vi "fft_tmp.vi"() -> ()   [LabVIEW 2014]
uses:
  <vilib>/express/express analysis/Spectral/Block/exnSpectralBlock spectral measurements peak poly.vi
  <vilib>/express/express analysis/Spectral/Block/exnSpectralBlock spectral measurements peak WFM.vi
  <vilib>/express/express analysis/Spectral/XNode/ExpressSpectralMeasurementsBlockNode.xnode
panel:
  in  "array":dbl[](array[numeric])
  in  "fft_FILE PATH 3":path=path "D:/testdata_v6"
  in  "FILE NAME 4":string="v6_" caption="FFTFILE NAME 2"
  out "CUR_CHP 2":u8 caption="CHIP"
  out "CUR_CHN 2":u8=1 caption="CHANNEL"
  out "Waveform Graph 2":cluster{"f0":dbl, "df":dbl, "magnitude":dbl[]}(graph)={"f0"=0.0, "df"=199.98000199980004, "magnitude"=array[5001 elements]}
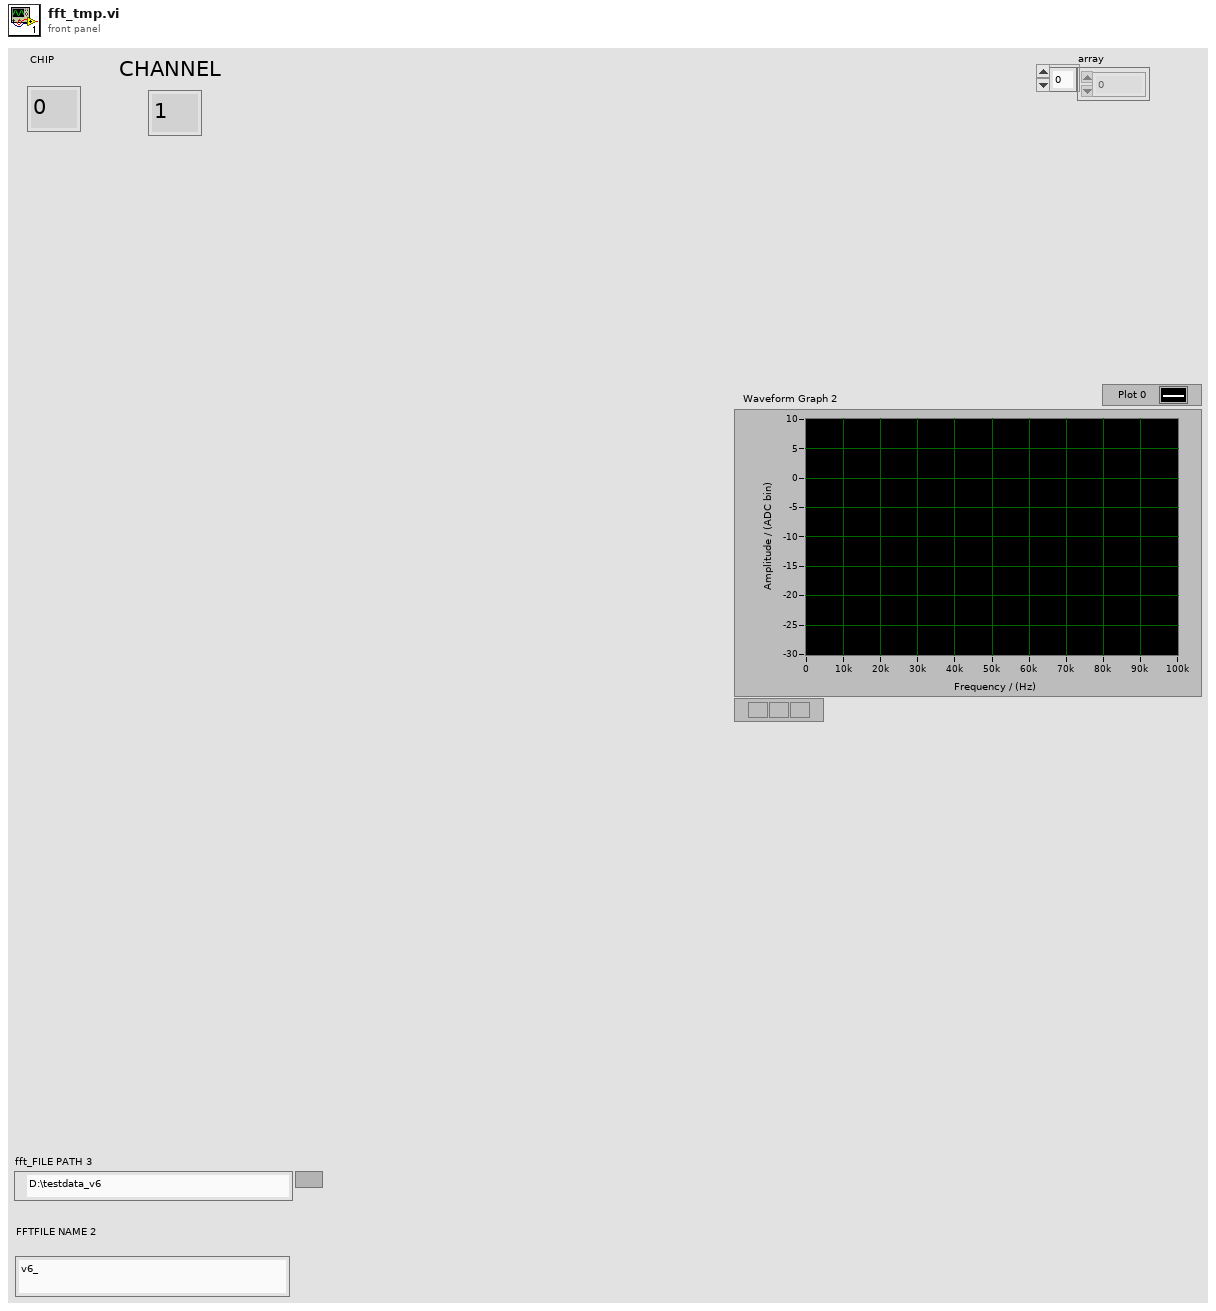
[diagram p1: front panel]
types:
  T1 = cluster{"averaging mode":u16, "weighting mode":u16, "number of averages":u32}
  T2 = cluster{"dB On (F)":bool, "unwrap phase (F)":bool, "convert to degree (F)":bool}
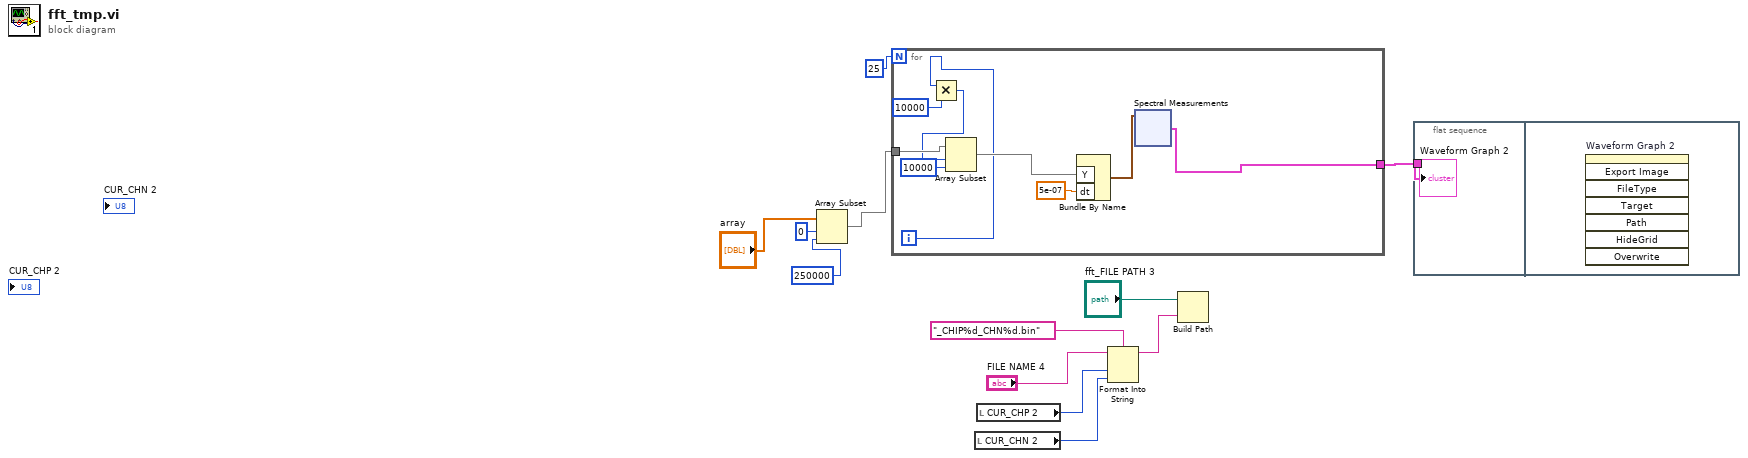
[diagram p0: block diagram]
diagram:
  n1 = Array Subset(array="array", index=0, length=250000) -> (w9:dbl[])
  n2 = for {
    N: 25 -> [_]
    tunnel: w9 -> [w21]
    tunnel: [w13] -> w8
    i -> [w14]
    n3 = Multiply(x=w14, y=10000) -> (x*y=w19:i32)
    n4 = Array Subset(array=w21, index=w19, length=10000) -> (w16:dbl[])
    n5 = Bundle By Name("Y"=w16, "dt"=5e-07) -> (w15:waveform(dbl))  [unwired: 1 in]
    n6 = xnode "Spectral Measurements"("Signals"=w15) -> ("FFT - (Peak)"=w13:cluster{"f0":dbl, "df":dbl, "magnitude":dbl[]})  [unwired: 2 in, 3 out]
  }
  n7 = local read "CUR_CHN 2"() -> (w2:u8)
  n8 = local read "CUR_CHP 2"() -> (w4:u8)
  n9 = Format Into String(format string="_CHIP%d_CHN%d.bin", initial string="FILE NAME 4", w4, w2) -> (resulting string=w6:string)  [unwired: 1 in, 1 out]
  n10 = Build Path(base path="fft_FILE PATH 3", name or relative path=w6) -> ()  [unwired: 1 out]
  n11 = flat-sequence {
    tunnel: w8 -> [w33]
    frame #0 {
      "Waveform Graph 2" <- w33
    }
    frame #1 {
      n12 = invoke on="Waveform Graph 2" class="WFGraph (strict)" method="Export Image"() -> ()  [unwired: 8 in, 8 out]
    }
  }
